vi "Viagogo Test.vi"() -> ()   [LabVIEW 2015]
panel:
  out "5":string
  out "4":string
  out "3":string
  out "2":string
  out "1":string
  out "Nearest Events":dbl[][](array[numeric])
  out "Event Info":dbl[][](array[numeric])
  out "Map":dbl[][][](array[numeric])
  # "Events closest to you:"
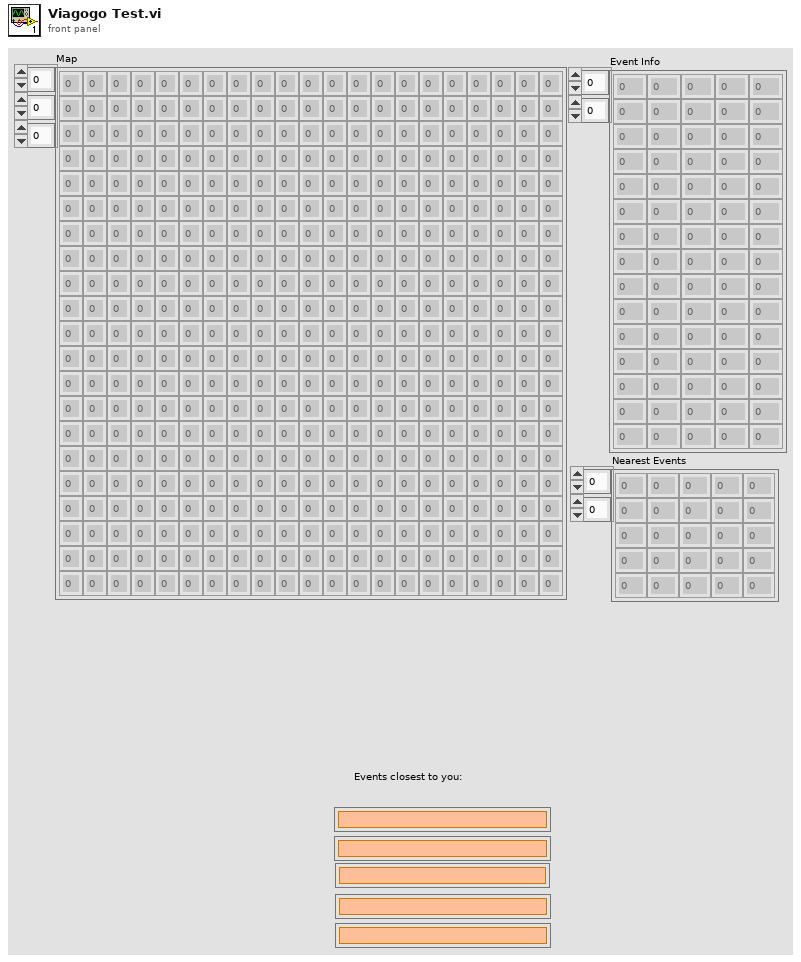
[diagram p1: front panel]
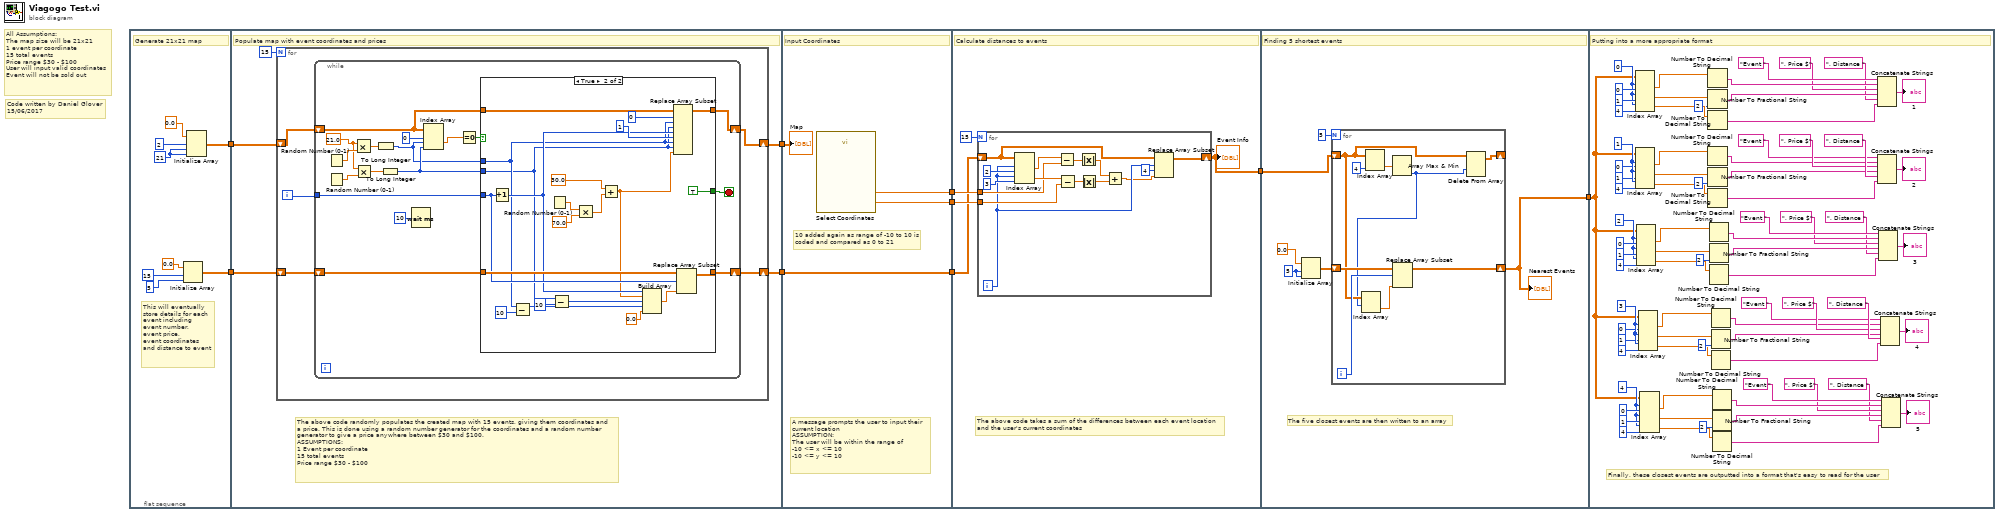
[diagram p0: block diagram]
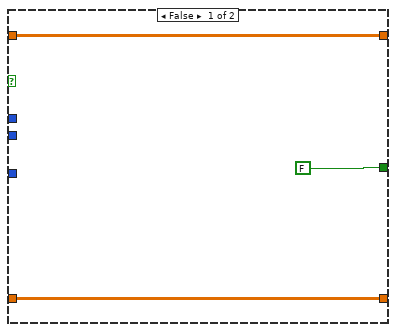
[diagram p2: hidden frame]
diagram:
  # "Code written by Daniel Glover\n15/06/2017"
  # "All Assumptions:\nThe map size will be 21x21\n1 event per coordinate\n15 total events\nPrice range $30 - $100\nUser will input valid coordinates\nEvent will not be sold out"
  n1 = flat-sequence {
    tunnel: [w16] -> w9
    tunnel: [w10] -> w7
    tunnel: w9 -> [w22]
    tunnel: [w20] -> w8
    tunnel: w7 -> [w19]
    tunnel: [w18] -> w6
    tunnel: w8 -> [w73]
    tunnel: w6 -> [w72]
    tunnel: [w72] -> w5
    tunnel: [w71] -> w4
    tunnel: [w70] -> w3
    tunnel: w5 -> [w75]
    tunnel: w4 -> [w77]
    tunnel: w3 -> [w76]
    tunnel: [w74] -> w2
    tunnel: w2 -> [w98]
    tunnel: [w94] -> w1
    tunnel: w1 -> [w113]
    frame #0 {
      w15 = 21 ("dimension size")
      # "This will eventually\nstore details for each\nevent including\nevent number,\nevent price,\nevent coordinates\nand distance to event"
      # "Generate 21x21 map"
      n2 = Initialize Array(0.0 ("element"), 15, 5) -> (w10:dbl[][])
      n3 = Initialize Array(0.0 ("element"), 2 ("dimension size"), w15, w15) -> (w16:dbl[][][])
    }
    frame #1 {
      # "The above code randomly populates the created map with 15 events, giving them coordinates and\na price. This is done using a random number generator for the coordinates and a random number\ngenerator to give a price anywhere between $30 and $100.\nASSUMPTIONS:\n1 Event per coordinate\n15 total events\nPrice range $30 - $100"
      # "Populate map with event coordinates and prices"
      n4 = for {
        N: 15 -> [_]
        shift-right: [w26] -> w20
        shift-left: w22 -> [w27]
        shift-right: [w23] -> w18
        shift-left: w19 -> [w25]
        i -> [w24]
        n5 = while {
          tunnel: w24 -> [w31]
          shift-right: [w34] -> w26
          shift-left: w27 -> [w36]
          shift-right: [w28] -> w23
          shift-left: w25 -> [w29]
          stop <- w35 stop-if-true
          w41 = 21.0 ("element")
          n6 = Random Number (0-1)() -> (number: 0 to 1=w43:dbl)
          n7 = Random Number (0-1)() -> (number: 0 to 1=w42:dbl)
          n8 = Multiply(x=w41, y=w43) -> (x*y=w40:dbl)
          n9 = Multiply(x=w41, y=w42) -> (x*y=w39:dbl)
          n10 = To Long Integer(number=w40) -> (32bit integer=w32:i32)
          n11 = To Long Integer(number=w39) -> (32bit integer=w33:i32)
          n12 = Wait (ms)(milliseconds to wait=u32 10) -> ()  [unwired: 1 out]
          n13 = Index Array(array=w36, index (dim 0)=0 ("dimension size"), index (dim 1)=w32, index (dim 2)=w33) -> (element=w37:dbl)
          n14 = Equal To 0?(x=w37) -> (x = 0?=w38:bool)
          n15 = case shown="True" w38 {
            tunnel: w36 -> [w47 w69]
            tunnel: [FALSE TRUE] -> w35
            tunnel: [w47 w67] -> w34
            tunnel: w33 -> [_ w49]
            tunnel: w32 -> [_ w54]
            tunnel: w31 -> [_ w59]
            tunnel: w29 -> [w45 w60]
            tunnel: [w45 w58] -> w28
            frame False {
            }
            frame True {
              n16 = Increment(x=w59) -> (x+1=w56:i32)
              n17 = Subtract(x=w54, y=10) -> (x-y=w52:i32)
              n18 = Random Number (0-1)() -> (number: 0 to 1=w64:dbl)
              n19 = Subtract(x=w49, y=10) -> (x-y=w50:i32)
              n20 = Multiply(x=w64, y=70.0) -> (x*y=w62:dbl)
              n21 = Add(x=30.0, y=w62) -> (x+y=w55:dbl)
              n22 = Build Array(w56, w55, w50, w52, 0.0 ("element")) -> (w57:dbl[])
              n23 = Replace Array Subset(array=w69, new element #1=w56, index (dim 0) #1=0 ("disabled index (page)"), index (dim 1) #1=w54, index (dim 2) #1=w49, new element #2=w55, index (dim 0) #2=1 ("disabled index (page)"), index (dim 1) #2=w54, index (dim 2) #2=w49) -> (w67:dbl[][][])
              n24 = Replace Array Subset(array=w60, new element=w57, index (row)=w59) -> (w58:dbl[][])  [unwired: 1 in]
            }
          }
        }
      }
    }
    frame #2 {
      # "10 added again as range of -10 to 10 is\ncoded and compared as 0 to 21"
      # "A message prompts the user to input their\ncurrent location\nASSUMPTION:\nThe user will be within the range of\n-10 <= x <= 10\n-10 <= y <= 10"
      # "Input Coordinates"
      n25 = call "Select Coordinates"() -> ("Input Y Coordinate"=w70:dbl, "Input X Coordinate"=w71:dbl)  [unwired: 16 in, 2 out]
      "Map" <- w73
    }
    frame #3 {
      # "The above code takes a sum of the differences between each event location\nand the user's current coordinates"
      # "Calculate distances to events"
      n26 = for {
        N: 15 -> [_]
        tunnel: w77 -> [w89]
        tunnel: w76 -> [w88]
        shift-right: [w82] -> w74
        shift-left: w75 -> [w83]
        i -> [w81]
        n27 = Index Array(array=w83, index (row) #1=w81, index (col) #1=2 ("dimension size"), index (row) #2=w81, index (col) #2=3 ("dimension size")) -> (element #1=w91:dbl, element #2=w90:dbl)
        n28 = Subtract(x=w91, y=w89) -> (x-y=w87:dbl)
        n29 = Subtract(x=w90, y=w88) -> (x-y=w86:dbl)
        n30 = Absolute Value(x=w87) -> (abs(x)=w85:dbl)
        n31 = Absolute Value(x=w86) -> (abs(x)=w84:dbl)
        n32 = Add(x=w85, y=w84) -> (x+y=w79:dbl)
        n33 = Replace Array Subset(array=w83, new element=w79, index (row)=w81, index (col)=4 ("disabled index (col)")) -> (w82:dbl[][])
      }
      "Event Info" <- w74
    }
    frame #4 {
      w97 = 5 ("dimension size")
      # "The five closest events are then written to an array"
      # "Finding 5 shortest events"
      n34 = Initialize Array(0.0 ("element"), w97, w97) -> (w95:dbl[][])
      n35 = for {
        N: 5 -> [_]
        shift-right: [w100] -> _
        shift-left: w98 -> [w102]
        shift-right: [w103] -> w94
        shift-left: w95 -> [w106]
        i -> [w105]
        n36 = Index Array(array=w102, index (col)=4 ("disabled index (col)")) -> (element=w107:dbl[])  [unwired: 1 in]
        n37 = Array Max & Min(array=w107) -> (min index (indices)=w101:i32)  [unwired: 3 out]
        n38 = Index Array(array=w102, index (row)=w101) -> (element=w104:dbl[])  [unwired: 1 in]
        n39 = Replace Array Subset(array=w106, new element=w104, index (row)=w105) -> (w103:dbl[][])  [unwired: 1 in]
        n40 = Delete From Array(array=w102, index (row)=w101) -> (array with subset deleted=w100:dbl[][])  [unwired: 2 in, 1 out]
      }
      "Nearest Events" <- w94
    }
    frame #5 {
      w124 = 4 ("index (row)")
      w131 = 3 ("index (row)")
      w152 = 2 ("index (row)")
      w159 = 1 ("index (row)")
      w181 = 0 ("index (row)")
      # "Finally, these closest events are outputted into a format that's easy to read for the user"
      # "Putting into a more appropriate format"
      n41 = Index Array(array=w113, index (row) #1=w181, index (col) #1=0 ("index (row)"), index (row) #2=w181, index (col) #2=1 ("index (row)"), index (row) #3=w181, index (col) #3=4 ("index (row)")) -> (element #1=w180:dbl, element #2=w179:dbl, element #3=w178:dbl)
      n42 = Index Array(array=w113, index (row) #1=w159, index (col) #1=0 ("index (row)"), index (row) #2=w159, index (col) #2=1 ("index (row)"), index (row) #3=w159, index (col) #3=4 ("index (row)")) -> (element #1=w160:dbl, element #2=w161:dbl, element #3=w162:dbl)
      n43 = Index Array(array=w113, index (row) #1=w152, index (col) #1=0 ("index (row)"), index (row) #2=w152, index (col) #2=1 ("index (row)"), index (row) #3=w152, index (col) #3=4 ("index (row)")) -> (element #1=w151:dbl, element #2=w150:dbl, element #3=w149:dbl)
      n44 = Index Array(array=w113, index (row) #1=w131, index (col) #1=0 ("index (row)"), index (row) #2=w131, index (col) #2=1 ("index (row)"), index (row) #3=w131, index (col) #3=4 ("index (row)")) -> (element #1=w132:dbl, element #2=w133:dbl, element #3=w134:dbl)
      n45 = Index Array(array=w113, index (row) #1=w124, index (col) #1=0 ("index (row)"), index (row) #2=w124, index (col) #2=1 ("index (row)"), index (row) #3=w124, index (col) #3=4 ("index (row)")) -> (element #1=w123:dbl, element #2=w122:dbl, element #3=w121:dbl)
      n46 = Number To Decimal String(number=w180) -> (decimal integer string=w176:string)  [unwired: 1 in]
      n47 = Number To Fractional String(number=w179, precision (6)=i16 2) -> (F-format string=w174:string)  [unwired: 2 in]
      n48 = Number To Decimal String(number=w178) -> (decimal integer string=w172:string)  [unwired: 1 in]
      n49 = Number To Decimal String(number=w160) -> (decimal integer string=w164:string)  [unwired: 1 in]
      n50 = Number To Fractional String(number=w161, precision (6)=i16 2) -> (F-format string=w166:string)  [unwired: 2 in]
      n51 = Number To Decimal String(number=w162) -> (decimal integer string=w168:string)  [unwired: 1 in]
      n52 = Number To Decimal String(number=w151) -> (decimal integer string=w147:string)  [unwired: 1 in]
      n53 = Number To Fractional String(number=w150, precision (6)=i16 2) -> (F-format string=w145:string)  [unwired: 2 in]
      n54 = Number To Decimal String(number=w149) -> (decimal integer string=w143:string)  [unwired: 1 in]
      n55 = Number To Decimal String(number=w132) -> (decimal integer string=w136:string)  [unwired: 1 in]
      n56 = Number To Fractional String(number=w133, precision (6)=i16 2) -> (F-format string=w138:string)  [unwired: 2 in]
      n57 = Number To Decimal String(number=w134) -> (decimal integer string=w140:string)  [unwired: 1 in]
      n58 = Number To Decimal String(number=w123) -> (decimal integer string=w119:string)  [unwired: 1 in]
      n59 = Number To Fractional String(number=w122, precision (6)=i16 2) -> (F-format string=w117:string)  [unwired: 2 in]
      n60 = Number To Decimal String(number=w121) -> (decimal integer string=w115:string)  [unwired: 1 in]
      n61 = Concatenate Strings("Event ", w176, ", Price $", w174, ", Distance ", w172) -> (→"1":string)
      n62 = Concatenate Strings("Event ", w164, ", Price $", w166, ", Distance ", w168) -> (→"2":string)
      n63 = Concatenate Strings("Event ", w147, ", Price $", w145, ", Distance ", w143) -> (→"3":string)
      n64 = Concatenate Strings("Event ", w136, ", Price $", w138, ", Distance ", w140) -> (→"4":string)
      n65 = Concatenate Strings("Event ", w119, ", Price $", w117, ", Distance ", w115) -> (→"5":string)
    }
  }
